vi "Record voice coil voltage vs input voltage.vi"() -> ()   [LabVIEW 2020]
uses:
  <vilib>/DAQmx/write.llb/DAQmx Write (Analog Wfm 1Chan NSamp).vi
  <vilib>/DAQmx/read.llb/DAQmx Read (Analog 1D DBL 1Chan NSamp).vi
  <vilib>/Utility/file.llb/Read Delimited Spreadsheet (DBL).vi
  <vilib>/DAQmx/create/channels.llb/DAQmx Create Channel (AI-Voltage-Basic).vi
  <vilib>/DAQmx/create/channels.llb/DAQmx Create Channel (AO-Voltage-Basic).vi
  <vilib>/DAQmx/configure/timing.llb/DAQmx Timing (Sample Clock).vi
  <vilib>/DAQmx/miscellaneous.llb/DAQmx Fill In Error Info.vi
  <vilib>/DAQmx/create/channels.llb/DAQmx Create Channel (CO-Pulse Generation-Frequency).vi
  <vilib>/DAQmx/configure/timing.llb/DAQmx Timing (Implicit).vi
  <resource>/objmgr/daqmx.rc
panel:
  out "data":dbl[](array[numeric])=[-0.16603452307496297, -0.15781252505752463, -0.16340348370047655, -0.1602791244541628, -0.15156380661897564, -0.16225240397677534, -0.16159464413538074, -0.16159464413538074, -0.15929248469462404, -0.15731920517908038, -0.1569903252602811, -0.1545237258734562, -0.1571547652196644, -0.1533726461621221, -0.1497549670797827, -0.11752473595178464, -0.14761724762946798, -0.1321598917681596, -0.16685672288121, -0.1522215664523896, -0.14876832733279782, -0.14498620831357784, -0.14679504784235467, -0.14531508822760716, -0.1430129288321425, -0.14432844848591073, -0.1497549670797827, -0.1407107694430711, -0.14087520939922138, -0.14268404891902667, -0.1405463294869534, -0.13906636988336127, -0.1416974091804619, -0.13824417010472867, -0.13561313081857848, -0.1786964001820755, -0.13281765158618003, -0.13298209154076654, -0.1430129288321425, -0.1315021319506599, -0.1315021319506599, -0.13298209154076654, -0.11127601781640872, -0.13396873126896916, -0.14153296922414857, -0.12443121394541111, -0.11999133522864647, -0.11078269796561016, -0.12262237446535192, -0.12410233403965334, -0.12476009385129884, -0.10338290023862047, -0.12147129479827017, -0.11900469551702521, -0.1609368842945099, -0.11653809624308475, -0.11736029600025352, -0.11538701658441132, -0.10601393942292556, -0.12212905460783625, -0.08973438460290956, -0.1132492972225206, -0.10749389896773974, -0.09960078142569619, -0.118346935709927, -0.10897385851517759, -0.10486285977877233, -0.10206738064957516, -0.09762750205183224, -0.10486285977877233, -0.1043695399317637, -0.10321846028987654, -0.1045339798807342, -0.1609368842945099, -0.09927190152972884, -0.08940550471081908, -0.09910746158179368, -0.0977919419994764, -0.09154322401171515, -0.09614754252448932, -0.10617837937221981, -0.09466758299976413, -0.09499646289392132, -0.09384538326493654, -0.09384538326493654, -0.040237962290930095, -0.09022770444128733, -0.10321846028987654, -0.0846367462900104, -0.08940550471081908, -0.09532534278820776, -0.07822358845650122, -0.08710334546980006, -0.09252986369089208, -0.08513006612538783, -0.08792554519800942, -0.08233458706208563, -0.08052574767314781, -0.08332122673042257, -0.0808546275617556] format="%0.2f"
  in  "file path (dialog if empty) 2":path=path "C:/Users/htm22/Downloads/Voice coil input.txt"
  out "actual frequency":dbl=10.0
  in  "stop":bool
  out "Signal input to voice coil (blue)":dbl[](graph)=[-0.285, -0.284, -0.284, -0.283, -0.282, -0.282, -0.281, -0.28, -0.28, -0.279, -0.278, -0.278, -0.277, -0.277, -0.276, -0.275, -0.275, -0.274, -0.273, -0.273, -0.272, -0.271, -0.271, -0.27, -0.269, -0.269, -0.268, -0.267, -0.267, -0.266, -0.266, -0.265, -0.264, -0.264, -0.263, -0.262, -0.262, -0.261, -0.26, -0.26, -0.259, -0.258, -0.258, -0.257, -0.257, -0.256, -0.255, -0.255, -0.254, -0.253, -0.253, -0.252, -0.251, -0.251, -0.25, -0.25, -0.249, -0.248, -0.248, -0.247, -0.246, -0.246, -0.245, -0.244, -0.244, -0.243, -0.243, -0.242, -0.241, -0.241, -0.24, -0.239, -0.239, -0.238, -0.237, -0.237, -0.236, -0.236, -0.235, -0.234, -0.234, -0.233, -0.232, -0.232, -0.231, -0.231, -0.23, -0.229, -0.229, -0.228, -0.227, -0.227, -0.226, -0.226, -0.225, -0.224, -0.224, -0.223, -0.222, -0.222, -0.221, -0.221, -0.22, -0.219, -0.219, -0.218, -0.218, -0.217, -0.216, -0.216, -0.215, -0.214, -0.214, -0.213, -0.213, -0.212, -0.211, -0.211, -0.21, -0.209, -0.209, -0.208, -0.208, -0.207, -0.206, -0.206, -0.205, -0.205, -0.204, -0.203, -0.203, -0.202, -0.202, -0.201, -0.2, -0.2, -0.199, -0.198, -0.198, -0.197, -0.197, -0.196, -0.195, -0.195, -0.194, -0.194, -0.193, -0.192, -0.192, -0.191, -0.191, -0.19, -0.189, -0.189, -0.188, -0.188, -0.187, -0.186, -0.186, -0.185, -0.185, -0.184, -0.183, -0.183, -0.182, -0.182, -0.181, -0.18, -0.18, -0.179, -0.179, -0.178, -0.177, -0.177, -0.176, -0.176, -0.175, -0.174, -0.174, -0.173, -0.173, -0.172, -0.171, -0.171, -0.17, -0.17, -0.169, -0.168, -0.168, -0.167, -0.167, -0.166, -0.165, -0.165, -0.164, -0.164, -0.163, -0.162, -0.162, -0.161, -0.161, -0.16, -0.16, -0.159, -0.158, -0.158, -0.157, -0.157, -0.156, -0.155, -0.155, -0.154, -0.154, -0.153, -0.153, -0.152, -0.151, -0.151, -0.15, -0.15, -0.149, -0.148, -0.148, -0.147, -0.147, -0.146, -0.146, -0.145, -0.144, -0.144, -0.143, -0.143, -0.142, -0.141, -0.141, -0.14, -0.14, -0.139, -0.139, -0.138, -0.137, -0.137, -0.136, -0.136, -0.135, -0.135, -0.134, -0.133, -0.133, -0.132, -0.132, -0.131, -0.131, -0.13, -0.129, -0.129, -0.128, -0.128, -0.127, -0.127, -0.126, -0.125, -0.125, -0.124, -0.124, -0.123, -0.123, -0.122, -0.121, -0.121, -0.12, -0.12, -0.119, -0.119, -0.118, -0.117, -0.117, -0.116, -0.116, -0.115, -0.115, -0.114, -0.114, -0.113, -0.112, -0.112, -0.111, -0.111, -0.11, -0.11, -0.109, -0.108, -0.108, -0.107, -0.107, -0.106, -0.106, -0.105, -0.105, -0.104, -0.103, -0.103, -0.102, -0.102, -0.101, -0.101, -0.1, -0.1, -0.099, -0.098, -0.098, -0.097, -0.097, -0.096, -0.096, -0.095, -0.095, -0.094, -0.094, -0.093, -0.092, -0.092, -0.091, -0.091, -0.09, -0.09, -0.089, -0.089, -0.088, -0.087, -0.087, -0.086, -0.086, -0.085, -0.085, -0.084, -0.084, -0.083, -0.083, -0.082, -0.081, -0.081, -0.08, -0.08, -0.079, -0.079, -0.078, -0.078, -0.077, -0.077, -0.076, -0.076, -0.075, -0.074, -0.074, -0.073, -0.073, -0.072, -0.072, -0.071, -0.071, -0.07, -0.07, -0.069, -0.069, -0.068, -0.067, -0.067, -0.066, -0.066, -0.065, -0.065, -0.064, -0.064, -0.063, -0.063, -0.062, -0.062, -0.061, -0.061, -0.06, -0.059, -0.059, -0.058, -0.058, -0.057, -0.057, -0.056, -0.056, -0.055, -0.055, -0.054, -0.054, -0.053, -0.053, -0.052, -0.052, -0.051, -0.051, -0.05, -0.049, -0.049, -0.048, -0.048, -0.047, -0.047, -0.046, -0.046, -0.045, -0.045, -0.044, -0.044, -0.043, -0.043, -0.042, -0.042, -0.041, -0.041, -0.04, -0.04, -0.039, -0.039, -0.038, -0.038, -0.037, -0.036, -0.036, -0.035, -0.035, -0.034, -0.034, -0.033, -0.033, -0.032, -0.032, -0.031, -0.031, -0.03, -0.03, -0.029, -0.029, -0.028, -0.028, -0.027, -0.027, -0.026, -0.026, -0.025, -0.025, -0.024, -0.024, -0.023, -0.023, -0.022, -0.022, -0.021, -0.021, -0.02, -0.02, -0.019, -0.019, -0.018, -0.018, -0.017, -0.017, -0.016, -0.016, -0.015, -0.015, -0.014, -0.014, -0.013, -0.013, -0.012, -0.012, -0.011, -0.011, -0.01, -0.01, -0.009, -0.009, -0.008, -0.008, -0.007, -0.007, -0.006, -0.006, -0.005, -0.005, -0.004, -0.004, -0.003, -0.003, -0.002, -0.002, -0.001, -0.001, 0.0, 0.0, 0.001, 0.001, 0.002, 0.002, 0.003, 0.003, 0.004, 0.004, 0.005, 0.005, 0.006, 0.006, 0.007, 0.007, 0.008, 0.008, 0.009, 0.009, 0.01, 0.01, 0.011, 0.011, 0.011, 0.012, 0.012, 0.013, 0.013, 0.014, 0.014, 0.015, 0.015, 0.016, 0.016, 0.017, 0.017, 0.018, 0.018, 0.019, 0.019, 0.02, 0.02, 0.021, 0.021, 0.022, 0.022, 0.023, 0.023, 0.023, 0.024, 0.024, 0.025, 0.025, 0.026, 0.026, 0.027, 0.027, 0.028, 0.028, 0.029, 0.029, 0.03, 0.03, 0.031, 0.031, 0.032, 0.032, 0.032, 0.033, 0.033, 0.034, 0.034, 0.035, 0.035, 0.036, 0.036, 0.037, 0.037, 0.038, 0.038, 0.039, 0.039, 0.039, 0.04, 0.04, 0.041, 0.041, 0.042, 0.042, 0.043, 0.043, 0.044, 0.044, 0.045, 0.045, 0.046, 0.046, 0.046, 0.047, 0.047, 0.048, 0.048, 0.049, 0.049, 0.05, 0.05, 0.051, 0.051, 0.051, 0.052, 0.052, 0.053, 0.053, 0.054, 0.054, 0.055, 0.055, 0.056, 0.056, 0.056, 0.057, 0.057, 0.058, 0.058, 0.059, 0.059, 0.06, 0.06, 0.061, 0.061, 0.061, 0.062, 0.062, 0.063, 0.063, 0.064, 0.064, 0.065, 0.065, 0.065, 0.066, 0.066, 0.067, 0.067, 0.068, 0.068, 0.069, 0.069, 0.069, 0.07, 0.07, 0.071, 0.071, 0.072, 0.072, 0.073, 0.073, 0.073, 0.074, 0.074, 0.075, 0.075, 0.076, 0.076, 0.077, 0.077, 0.077, 0.078, 0.078, 0.079, 0.079, 0.08, 0.08, 0.08, 0.081, 0.081, 0.082, 0.082, 0.083, 0.083, 0.083, 0.084, 0.084, 0.085, 0.085, 0.086, 0.086, 0.087, 0.087, 0.087, 0.088, 0.088, 0.089, 0.089, 0.09, 0.09, 0.09, 0.091, 0.091, 0.092, 0.092, 0.093, 0.093, 0.093, 0.094, 0.094, 0.095, 0.095, 0.095, 0.096, 0.096, 0.097, 0.097, 0.098, 0.098, 0.098, 0.099, 0.099, 0.1, 0.1, 0.101, 0.101, 0.101, 0.102, 0.102, 0.103, 0.103, 0.103, 0.104, 0.104, 0.105, 0.105, 0.106, 0.106, 0.106, 0.107, 0.107, 0.108, 0.108, 0.108, 0.109, 0.109, 0.11, 0.11, 0.111, 0.111, 0.111, 0.112, 0.112, 0.113, 0.113, 0.113, 0.114, 0.114, 0.115, 0.115, 0.115, 0.116, 0.116, 0.117, 0.117, 0.117, 0.118, 0.118, 0.119, 0.119, 0.12, 0.12, 0.12, 0.121, 0.121, 0.122, 0.122, 0.122, 0.123, 0.123, 0.124, 0.124, 0.124, 0.125, 0.125, 0.126, 0.126, 0.126, 0.127, 0.127, 0.128, 0.128, 0.128, 0.129, 0.129, 0.13, 0.13, 0.13, 0.131, 0.131, 0.132, 0.132, 0.132, 0.133, 0.133, 0.133, 0.134, 0.134, 0.135, 0.135, 0.135, 0.136, 0.136, 0.137, 0.137, 0.137, 0.138, 0.138, 0.139, 0.139, 0.139, 0.14, 0.14, 0.141, 0.141, 0.141, 0.142, 0.142, 0.142, 0.143, 0.143, 0.144, 0.144, 0.144, 0.145, 0.145, 0.146, 0.146, 0.146, 0.147, 0.147, 0.147, 0.148, 0.148, 0.149, 0.149, 0.149, 0.15, 0.15, 0.15, 0.151, 0.151, 0.152, 0.152, 0.152, 0.153, 0.153, 0.154, 0.154, 0.154, 0.155, 0.155, 0.155, 0.156, 0.156, 0.157, 0.157, 0.157, 0.158, 0.158, 0.158, 0.159, 0.159, 0.159, 0.16, 0.16, 0.161, 0.161, 0.161, 0.162, 0.162, 0.162, 0.163, 0.163, 0.164, 0.164, 0.164, 0.165, 0.165, 0.165, 0.166, 0.166, 0.166, 0.167, 0.167, 0.168, 0.168, 0.168, 0.169, 0.169, 0.169, 0.17, 0.17, 0.17, 0.171, 0.171, 0.172, 0.172, 0.172, 0.173, 0.173, 0.173, 0.174, 0.174, 0.174, 0.175, 0.175, 0.176, 0.176, 0.176, 0.177, 0.177, 0.177, 0.178, 0.178, 0.178, 0.179, 0.179, 0.179, 0.18, 0.18, 0.18, 0.181, 0.181, 0.182, 0.182, 0.182, 0.183, 0.183, 0.183, 0.184, 0.184, 0.184, 0.185, 0.185, 0.185, 0.186, 0.186, 0.186, 0.187, 0.187, 0.187, 0.188, 0.188, 0.189, 0.189, 0.189, 0.19, 0.19, 0.19, 0.191, 0.191, 0.191, 0.192, 0.192, 0.192, 0.193, 0.193, 0.193, 0.194, 0.194, 0.194, 0.195, 0.195, 0.195, 0.196, 0.196, 0.196, 0.197, 0.197, 0.197, 0.198, 0.198, 0.198, 0.199, 0.199, 0.199, 0.2, 0.2, 0.2, 0.201, 0.201, 0.201, 0.202, 0.202, 0.202, 0.203, 0.203, 0.203, 0.204, 0.204, 0.204, 0.205, 0.205, 0.205, 0.206]
  out "# Samples written per channel":u32=1000
  out "Signal Output":dbl[](graph)=[-0.16603452307496297, -0.15781252505752463, -0.16340348370047655, -0.1602791244541628, -0.15156380661897564, -0.16225240397677534, -0.16159464413538074, -0.16159464413538074, -0.15929248469462404, -0.15731920517908038, -0.1569903252602811, -0.1545237258734562, -0.1571547652196644, -0.1533726461621221, -0.1497549670797827, -0.11752473595178464, -0.14761724762946798, -0.1321598917681596, -0.16685672288121, -0.1522215664523896, -0.14876832733279782, -0.14498620831357784, -0.14679504784235467, -0.14531508822760716, -0.1430129288321425, -0.14432844848591073, -0.1497549670797827, -0.1407107694430711, -0.14087520939922138, -0.14268404891902667, -0.1405463294869534, -0.13906636988336127, -0.1416974091804619, -0.13824417010472867, -0.13561313081857848, -0.1786964001820755, -0.13281765158618003, -0.13298209154076654, -0.1430129288321425, -0.1315021319506599, -0.1315021319506599, -0.13298209154076654, -0.11127601781640872, -0.13396873126896916, -0.14153296922414857, -0.12443121394541111, -0.11999133522864647, -0.11078269796561016, -0.12262237446535192, -0.12410233403965334, -0.12476009385129884, -0.10338290023862047, -0.12147129479827017, -0.11900469551702521, -0.1609368842945099, -0.11653809624308475, -0.11736029600025352, -0.11538701658441132, -0.10601393942292556, -0.12212905460783625, -0.08973438460290956, -0.1132492972225206, -0.10749389896773974, -0.09960078142569619, -0.118346935709927, -0.10897385851517759, -0.10486285977877233, -0.10206738064957516, -0.09762750205183224, -0.10486285977877233, -0.1043695399317637, -0.10321846028987654, -0.1045339798807342, -0.1609368842945099, -0.09927190152972884, -0.08940550471081908, -0.09910746158179368, -0.0977919419994764, -0.09154322401171515, -0.09614754252448932, -0.10617837937221981, -0.09466758299976413, -0.09499646289392132, -0.09384538326493654, -0.09384538326493654, -0.040237962290930095, -0.09022770444128733, -0.10321846028987654, -0.0846367462900104, -0.08940550471081908, -0.09532534278820776, -0.07822358845650122, -0.08710334546980006, -0.09252986369089208, -0.08513006612538783, -0.08792554519800942, -0.08233458706208563, -0.08052574767314781, -0.08332122673042257, -0.0808546275617556]
  in  "stop 2":bool
  out "Saving Data":bool
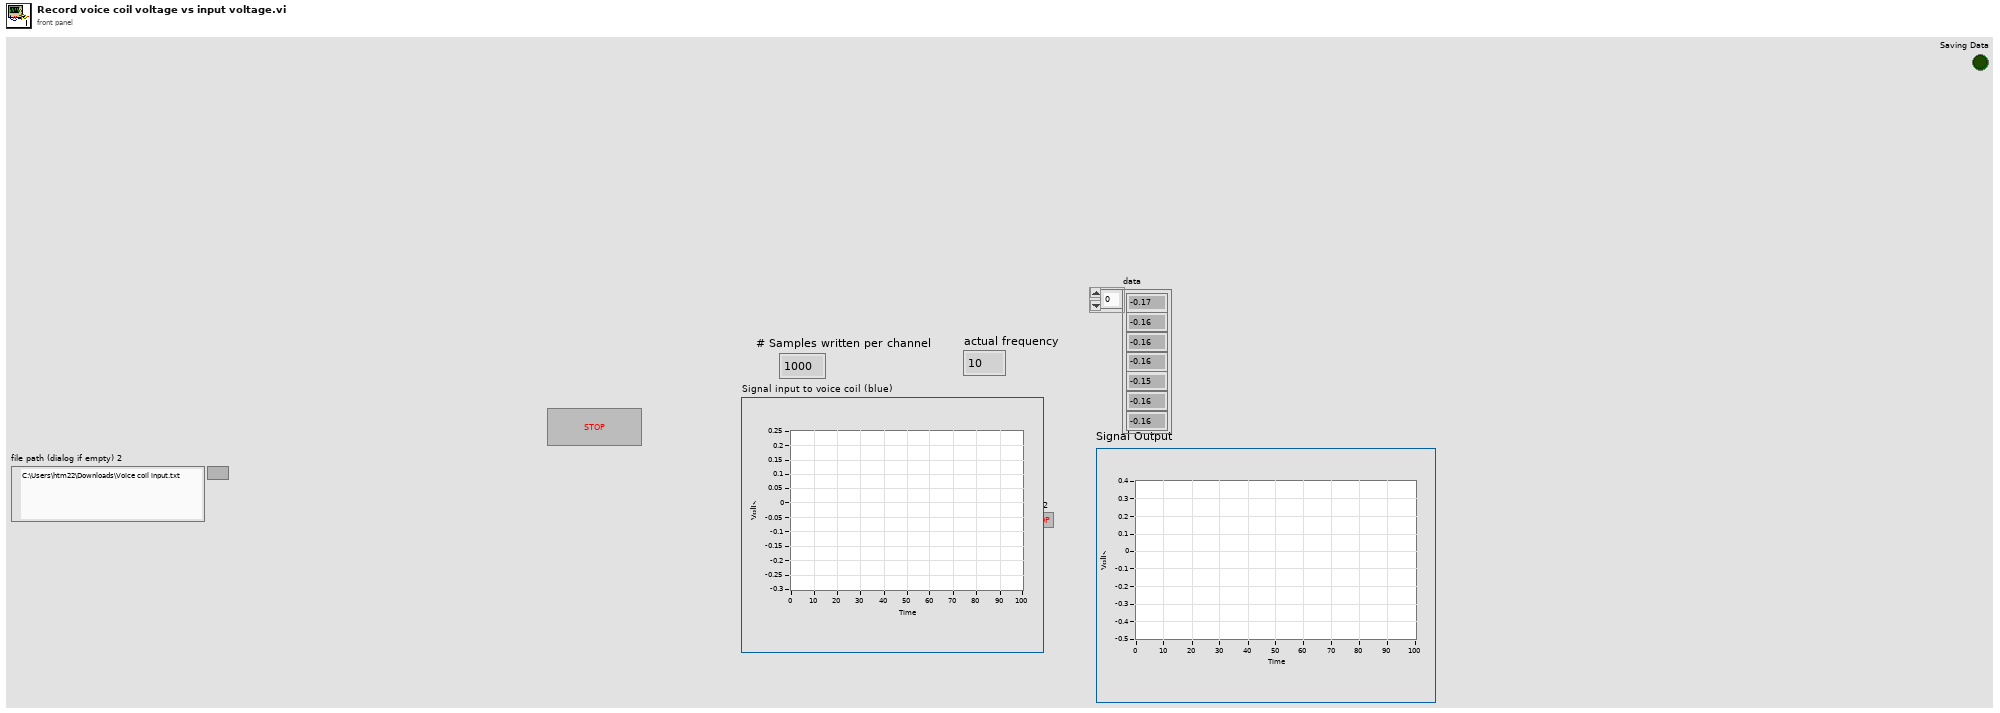
[diagram p1: front panel]
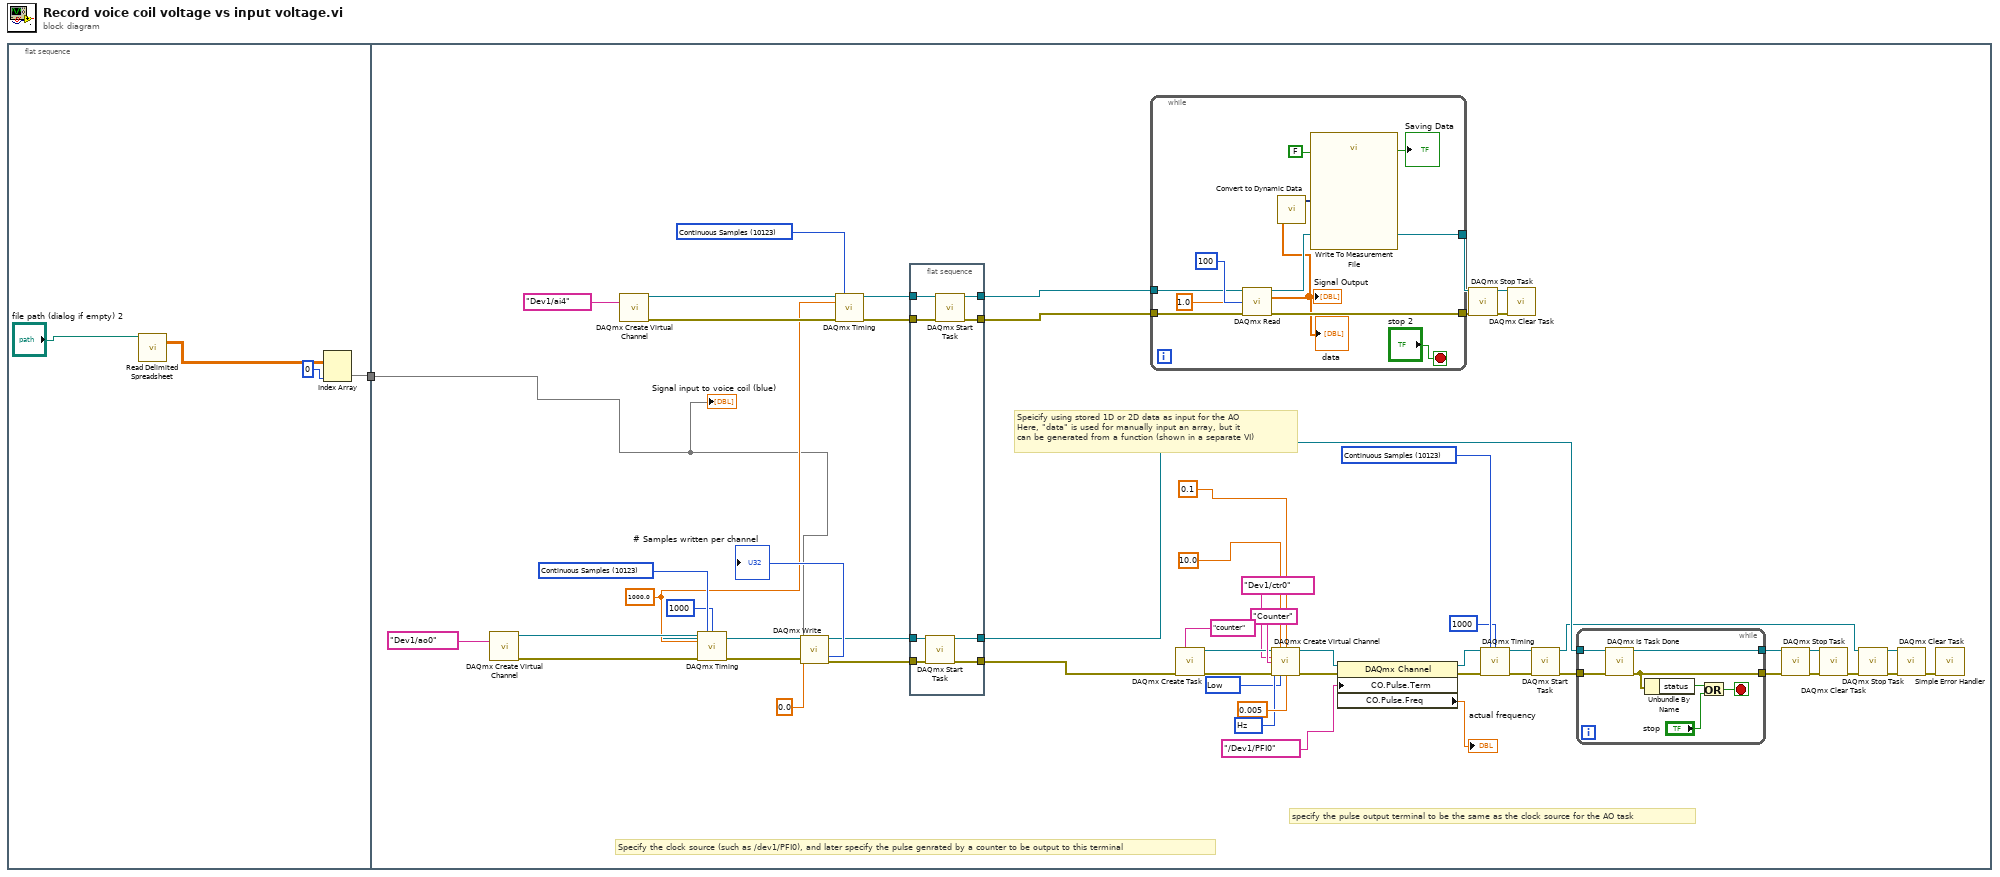
[diagram p0: block diagram]
diagram:
  n1 = flat-sequence {
    tunnel: [w3] -> w1
    tunnel: w1 -> [w8]
    frame #0 {
      n2 = call-poly <vilib>:"Read Delimited Spreadsheet.vi"("file path (dialog if empty)"="file path (dialog if empty) 2") -> ("all rows"=w2:dbl[][])  [unwired: 9 in, 5 out]
      n3 = Index Array(array=w2, index (col)=0 ("disabled index (col)")) -> (element=w3:dbl[])  [unwired: 1 in]
    }
    frame #1 {
      w11 = 10214 items=["High"=10192, "Low"=10214] ("idle state")
      w12 = 10373 items=["Hz"=10373] ("units")
      w44 = 10123 items=["Finite Samples"=10178, "Continuous Samples"=10123, "Hardware Timed Single Point"=12522] ("sample mode")
      w9 = 1000.0 ("rate")
      w48 = 10123 items=["Finite Samples"=10178, "Continuous Samples"=10123, "Hardware Timed Single Point"=12522] ("sample mode")
      w59 = 10123 items=["Finite Samples"=10178, "Continuous Samples"=10123, "Hardware Timed Single Point"=12522] ("sample mode")
      # "specify the pulse output terminal to be the same as the clock source for the AO task"
      # "Speicify using stored 1D or 2D data as input for the AO\nHere, \"data\" is used for manually input an array, but it\ncan be generated from a function (shown in a separate VI)"
      # "Specify the clock source (such as /dev1/PFI0), and later specify the pulse genrated by a counter to be output to this terminal"
      n4 = call-poly <vilib>:"DAQmx Create Virtual Channel.vi"("physical channels"=tag "Dev1/ao0") -> ("task out"=w50:refnum<k21>, "error out"=w49:errorcluster)  [unwired: 13 in]
      n5 = call-poly <vilib>:"DAQmx Create Virtual Channel.vi"("physical channels"=tag "Dev1/ai4") -> ("task out"=w62:refnum<k21>, "error out"=w61:errorcluster)  [unwired: 13 in]
      n6 = call-poly <vilib>:"DAQmx Timing.vi"("task/channels in"=w50, "sample mode"=w48, "samples per channel"=1000, "rate"=w9, "error in"=w49) -> ("task out"=w7:refnum<k21>, "error out"=w6:errorcluster)  [unwired: 9 in]
      n7 = call-poly <vilib>:"DAQmx Write.vi"("task/channels in"=w7, "data"=w8, "timeout"=0.0, "error in"=w6) -> ("task out"=w21:refnum<k21>, "number of samples written per channel"=→"# Samples written per channel":u32, "error out"=w20:errorcluster)  [unwired: 9 in]
      n8 = call-poly <vilib>:"DAQmx Timing.vi"("task/channels in"=w62, "sample mode"=w59, "rate"=w9, "error in"=w61) -> ("task out"=w58:refnum<k21>, "error out"=w57:errorcluster)  [unwired: 10 in]
      n9 = flat-sequence {
        tunnel: w58 -> [w70]
        tunnel: w57 -> [w69]
        tunnel: [w68] -> w54
        tunnel: [w67] -> w53
        tunnel: [w66] -> w45
        tunnel: [w65] -> w23
        tunnel: w21 -> [w64]
        tunnel: w20 -> [w63]
        frame #0 {
          n10 = call <vilib>:"DAQmx Start Task.vi"("task/channels in"=w64, "error in"=w63) -> ("task out"=w66:refnum<k21>, "error out"=w65:errorcluster)  [unwired: 12 in]
          n11 = call <vilib>:"DAQmx Start Task.vi"("task/channels in"=w70, "error in"=w69) -> ("task out"=w68:refnum<k21>, "error out"=w67:errorcluster)  [unwired: 12 in]
        }
      }
      n12 = while {
        tunnel: w54 -> [w87]
        tunnel: w53 -> [w86]
        tunnel: [w85] -> w52
        tunnel: [w84] -> w51
        stop <- "stop 2" stop-if-true
        n13 = call-poly <vilib>:"DAQmx Read.vi"("task/channels in"=w87, "number of samples per channel"=100, "timeout"=1.0, "error in"=w86) -> ("task out"=w85:refnum<k21>, "data"=w78:dbl[], "error out"=w84:errorcluster)  [unwired: 9 in]
        "Signal Output" <- w78
        "data" <- w78
        n14 = call "Convert to Dynamic Data"("Array"=w78) -> ("Dynamic Data Type"=w82:dynamicdata)  [unwired: 3 in]
        n15 = call "Write To Measurement File"("Signals"=w82, "Enable"=FALSE) -> ("Saving Data"=→"Saving Data":bool)  [unwired: 15 in, 2 out]
      }
      n16 = call <vilib>:"DAQmx Create Task.vi"("new task name"="counter", "error in"=w23) -> ("task out"=w40:refnum<k21>, "error out"=w38:errorcluster)  [unwired: 12 in]
      n17 = call-poly <vilib>:"DAQmx Create Virtual Channel.vi"("task in"=w40, "frequency"=10.0, "duty cycle"=0.1, "counter"=tag "Dev1/ctr0", "name to assign"="Counter", "units"=w12, "error in"=w38, "idle state"=w11, "initial delay"=0.005) -> ("task out"=w37:refnum<k21>, "error out"=w36:errorcluster)  [unwired: 5 in]
      n18 = property class="DAQmx Channel"(reference=w37, error in=w36, "CO.Pulse.Term"=tag "/Dev1/PFI0") -> (reference out=w33:refnum<k21>, error out=w34:errorcluster, "CO.Pulse.Freq"=→"actual frequency":dbl)
      n19 = call <vilib>:"DAQmx Stop Task.vi"("task/channels in"=w52, "error in"=w51) -> ("task out"=w55:refnum<k21>, "error out"=w56:errorcluster)  [unwired: 12 in]
      n20 = call-poly <vilib>:"DAQmx Timing.vi"("task/channels in"=w33, "sample mode"=w44, "samples per channel"=1000, "error in"=w34) -> ("task out"=w43:refnum<k21>, "error out"=w42:errorcluster)  [unwired: 10 in]
      n21 = call <vilib>:"DAQmx Clear Task.vi"("task in"=w55, "error in"=w56) -> ()  [unwired: 13 in, 1 out]
      n22 = call <vilib>:"DAQmx Start Task.vi"("task/channels in"=w43, "error in"=w42) -> ("task out"=w32:refnum<k21>, "error out"=w22:errorcluster)  [unwired: 12 in]
      n23 = while {
        tunnel: w45 -> [w77]
        tunnel: w22 -> [w76]
        tunnel: [w75] -> w28
        tunnel: [w74] -> w29
        stop <- w71 stop-if-true
        n24 = call <vilib>:"DAQmx Is Task Done.vi"("task/channels in"=w77, "error in"=w76) -> ("task out"=w75:refnum<k21>, "error out"=w74:errorcluster)  [unwired: 11 in, 1 out]
        n25 = Unbundle By Name(w74) -> ("status"=w73:bool)
        n26 = Or(x=w73, y="stop") -> (x .or. y?=w71:bool)
      }
      n27 = call <vilib>:"DAQmx Stop Task.vi"("task/channels in"=w28, "error in"=w29) -> ("task out"=w27:refnum<k21>, "error out"=w26:errorcluster)  [unwired: 12 in]
      n28 = call <vilib>:"DAQmx Clear Task.vi"("task in"=w27, "error in"=w26) -> ("error out"=w25:errorcluster)  [unwired: 13 in]
      n29 = call <vilib>:"DAQmx Stop Task.vi"("task/channels in"=w32, "error in"=w25) -> ("task out"=w30:refnum<k21>, "error out"=w31:errorcluster)  [unwired: 12 in]
      n30 = call <vilib>:"DAQmx Clear Task.vi"("task in"=w30, "error in"=w31) -> ("error out"=w24:errorcluster)  [unwired: 13 in]
      n31 = call <vilib>:"Simple Error Handler.vi"("error in (no error)"=w24) -> ()  [unwired: 4 in, 5 out]
      "Signal input to voice coil (blue)" <- w8
    }
  }
